vi "string form troll.vi"(11 "String":string) -> (3 "Array":u32[](array[numeric]))   [LabVIEW 2023]
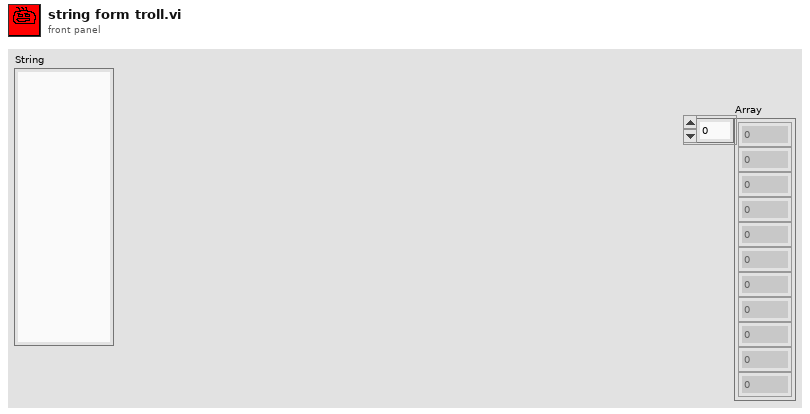
[diagram p1: front panel]
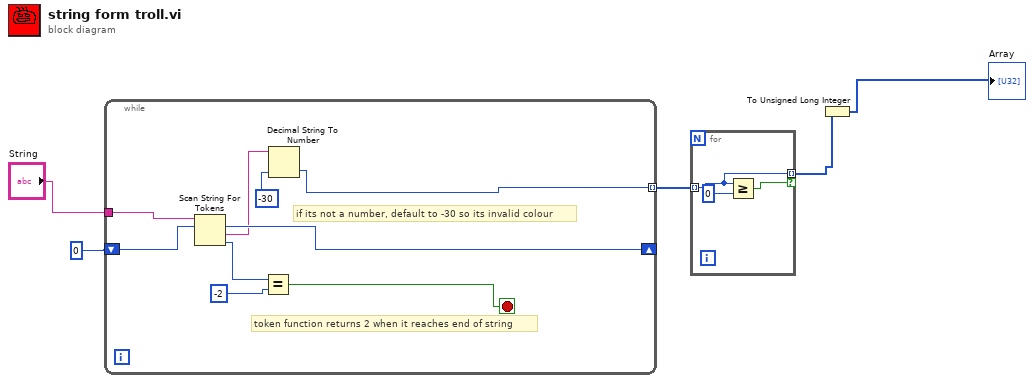
[diagram p0: block diagram]
diagram:
  n1 = while {
    shift-right: [w11] -> _
    shift-left: 0 ("offset past token") -> [w10]
    tunnel: "String" -> [w9]
    tunnel: [w6] -> w4 mode=indexing
    stop <- w13 stop-if-true
    # "token function returns 2 when it reaches end of string"
    # "if its not a number, default to -30 so its invalid colour"
    n2 = Scan String For Tokens(8:w10, 9:w9) -> (0:w14:i32, 1:w8:string, 2:w11:i32)  [unwired: 4 in, 1 out]
    n3 = Equal?(x=w14, y=-2) -> (x = y?=w13:bool)
    n4 = Decimal String To Number(string=w8, default (0L)=-30 ("default (0 I32)")) -> (number=w6:i32)  [unwired: 1 in, 1 out]
  }
  n5 = for {
    tunnel: w4 -> [w16] mode=indexing
    tunnel: [w16] -> w3 mode=indexing if=w15
    n6 = Greater Or Equal?(x=w16, y=0) -> (x >= y?=w15:bool)
  }
  n7 = To Unsigned Long Integer(number=w3) -> (unsigned 32bit integer=→"Array":u32[])
